vi "Initialize Hardware.vi"(8 "error in (no error)":errorcluster, 11 "Microscope_RM21 in":refnum<class "Microscope_RM21.lvclass">) -> (0 "error out":errorcluster, 3 "Microscope_RM21 out":refnum<class "Microscope_RM21.lvclass">)   [LabVIEW 2020, in "Microscope_RM21.lvlib" / "Microscope_RM21.lvclass"]
uses:
  Microscope_RM21.lvclass
  HAL Layer/Microscope/Microscope/Microscope.lvclass
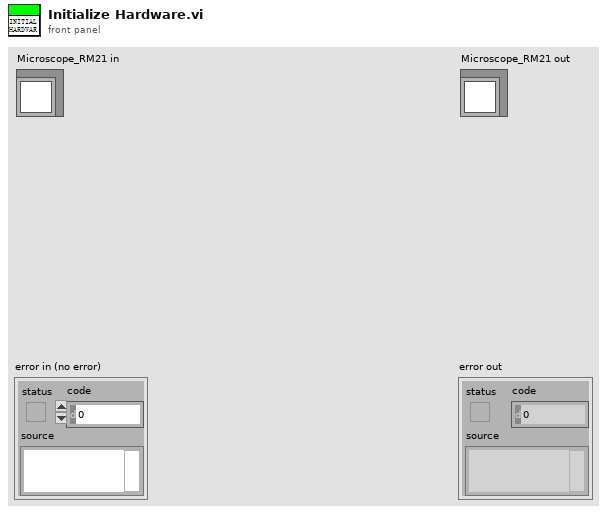
[diagram p1: front panel]
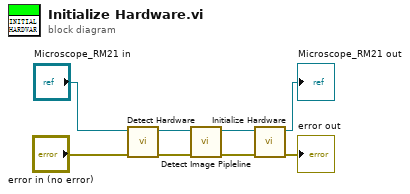
[diagram p0: block diagram]
diagram:
  n1 = call "Detect Hardware.vi"("error in (no error)"="error in (no error)", "Microscope_RM21 in"="Microscope_RM21 in") -> ("error out"=w5:errorcluster, "Microscope_RM21 out"=w2:refnum<class "Microscope_RM21.lvclass">)  [unwired: 8 in]
  n2 = call-dynamic "Detect Image Pipleline.vi"("error in (no error)"=w5, "Microscope_RM21 in"=w2) -> ("error out"=w3:errorcluster, "Microscope_RM21 out"=w1:refnum<class "Microscope_RM21.lvclass">)  [unwired: 8 in]
  n3 = call-parent "Initialize Hardware.vi"("error in (no error)"=w3, "Microscope in"=w1) -> ("error out"=→"error out":errorcluster, "Microscope out"=→"Microscope_RM21 out":refnum<class "Microscope_RM21.lvclass">)  [unwired: 8 in]
